vi "Create Dataset.vi"(7 "Dims meas":u64[](array[numeric]), 8 "error in (no error)":errorcluster, 9 "Variant":variant, 10 "Label.Text":string, 11 "Refnum in":T1) -> (0 "error out":errorcluster, 3 "Refnum out":T1)   [LabVIEW 2019]
uses:
  <vilib>/UPVI/lvhdf5/library.llb/HDF5 Ref.ctl
  <vilib>/Utility/Data Type/Type Definitions/Data Type.ctl
  <vilib>/UPVI/lvhdf5/property.llb/LVH5PClassId.ctl
  <vilib>/UPVI/lvhdf5/datatype.llb/LVH5Tcreate_element_type (Variant).vi
  <vilib>/UPVI/lvhdf5/datatype.llb/LVH5Tcreate_dataset_type (Variant).vi
  <vilib>/UPVI/lvhdf5/datatype.llb/LVH5Tcreate_element_type.xnode
  <vilib>/UPVI/lvhdf5/datatype.llb/LVH5Tcreate_dataset_type.xnode
  <vilib>/Utility/Data Type/NI_Data Type.lvlib
panel:
  out "Dims nat":u64[](array[numeric])
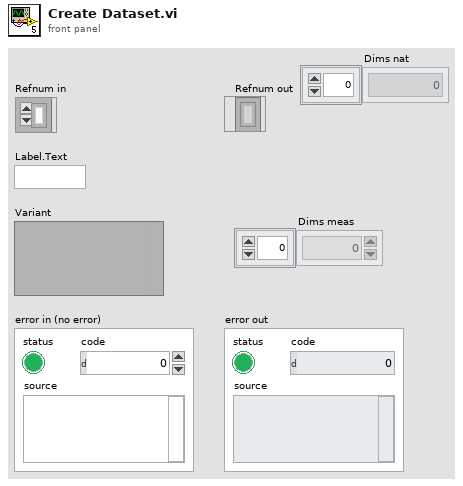
[diagram p1: front panel]
types:
  T1 = typedef "HDF5 Ref.ctl" = refnum<k1>
  T2 = typedef "LVH5PClassId.ctl" = enum32{"H5P_ROOT", "H5P_OBJECT_CREATE", "H5P_FILE_CREATE", "H5P_FILE_ACCESS", "H5P_DATASET_CREATE", "H5P_DATASET_ACCESS", "H5P_DATASET_XFER", "H5P_FILE_MOUNT", "H5P_GROUP_CREATE", "H5P_GROUP_ACCESS", "H5P_DATATYPE_CREATE", "H5P_DATATYPE_ACCESS", "H5P_STRING_CREATE", "H5P_ATTRIBUTE_CREATE", "H5P_OBJECT_COPY", "H5P_LINK_CREATE", "H5P_LINK_ACCESS"}
  T3 = typedef "NI_Data Type.lvlib/Data Type.ctl" = enum8{"Invalid Type", "Void", "I8", "I16", "I32", "I64", "U8", "U16", "U32", "U64", "Single Float", "Double Float", "Extended Float", "Single Complex", "Double Complex", "Extended Complex", "Enum U8", "Enum U16", "Enum U32", "Enum U64", "Single Float With Unit", "Double Float With Unit", "Extended Float With Unit", "Single Complex with Unit", "Double Complex with Unit", "Extended Complex with Unit", "Boolean", "String", "Path", "Picture", "Tag", "Array", "Cluster", "Variant", "LV Variant", "Waveform", "Timestamp", "Digital Waveform", "Digital Data", "ExpressData", "Refnum", "External Data", "VI", "Poly VI", "LabVIEW Class Instance", "Fixed Point", "Set Collection", "Map Collection"}
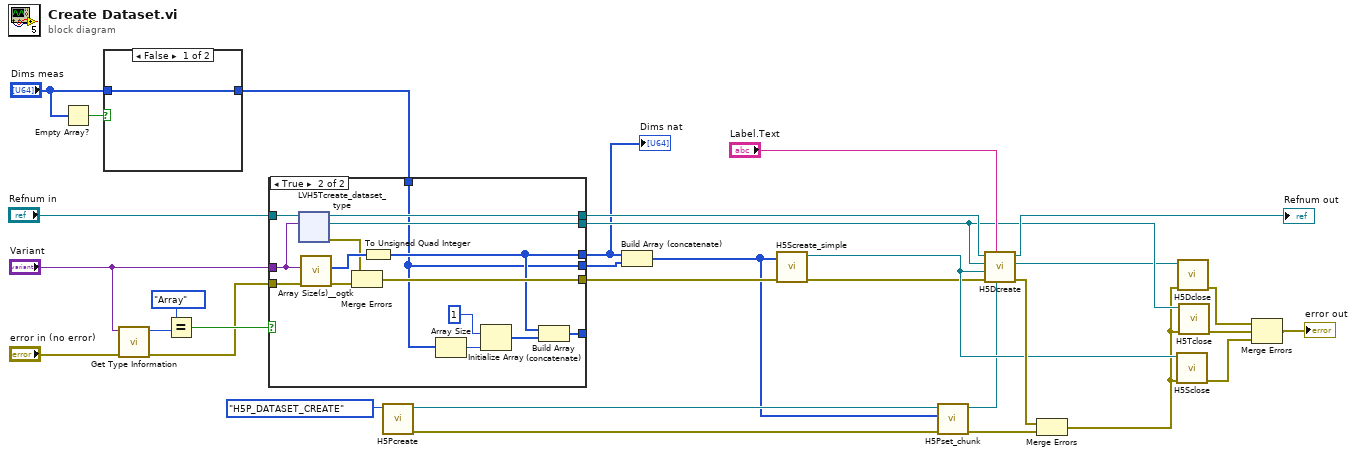
[diagram p0: block diagram]
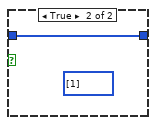
[diagram p2: hidden frame]
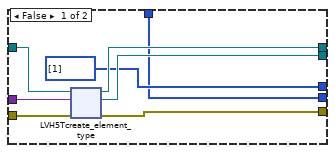
[diagram p3: hidden frame]
diagram:
  n1 = Empty Array?(array="Dims meas") -> (empty?=w4:bool)
  n2 = case shown="False" w4 {
    tunnel: "Dims meas" -> [w33 w34]
    tunnel: [w33 w34] -> w3
    frame False {
    }
    frame True {
      (unwired) u64[] [1] ("Dims meas")
    }
  }
  n3 = call <vilib>:"Get Type Information.vi"("error in (no error)"="error in (no error)", "variant"="Variant") -> ("error out"=w25:errorcluster, "type"=w30:T3)  [unwired: 5 in, 3 out]
  n4 = Equal?(x=Data_Type."Array", y=w30) -> (x = y?=w28:bool)
  n5 = case shown="True" w28 {
    tunnel: "Variant" -> [w37 w77]
    tunnel: w25 -> [w42 w81]
    tunnel: [u64[] [1] w72] -> w8
    tunnel: [w41 w76] -> w22
    tunnel: "Refnum in" -> [w40 w78]
    tunnel: [w38 w74] -> w20
    tunnel: [w39 w73] -> w23
    tunnel: [_ w71] -> _
    tunnel: w3 -> [w35 w67]
    tunnel: [w35 w67] -> w1
    frame False {
      n6 = xnode "LVH5Tcreate_element_type"("HDF5 Location Ref"=w40, "error in (no error)"=w42, "Data"=w37) -> ("HDF5 Location Ref out"=w39:T1, "HDF5 Type Ref"=w38:T1, "error out"=w41:errorcluster)  [unwired: 3 in, 2 out]
    }
    frame True {
      n7 = xnode "LVH5Tcreate_dataset_type"("HDF5 Location Ref"=w78, "Data"=w77) -> ("HDF5 Location Ref out"=w73:T1, "HDF5 Type Ref"=w74:T1, "error out"=w75:errorcluster)  [unwired: 4 in, 2 out]
      n8 = call <userlib>:"Array Size(s)__ogtk.vi"("error in (no error)"=w81, "Array"=w77) -> ("error out"=w79:errorcluster, "Size(s)"=w80:u32[])  [unwired: 7 in, 1 out]
      n9 = Merge Errors(w75, w79) -> (w76:errorcluster)
      n10 = To Unsigned Quad Integer(1:w80) -> (0:w72:u64[])
      n11 = Array Size(array=w67) -> (size(s)=w69:i32)
      n12 = Initialize Array(u64 1 ("element"), w69) -> (w70:u64[])
      n13 = Build Array (concatenate)(w72, w70) -> (w71:u64[])
    }
  }
  "Dims nat" <- w8
  n14 = call <vilib>:"H5Pcreate.vi"("Property List Class"=LVH5PClassId."H5P_DATASET_CREATE") -> ("error out"=w7:errorcluster, "HDF5 Property List Ref"=w6:T1)  [unwired: 7 in]
  n15 = Build Array (concatenate)(w8, w1) -> (w2:u64[])
  n16 = call <vilib>:"H5Screate_simple.vi"("error in (no error)"=w22, "Dimensions"=w2) -> ("error out"=w17:errorcluster, "HDF5 Ref out"=w18:T1)  [unwired: 6 in]
  n17 = call <vilib>:"H5Pset_chunk.vi"("error in (no error)"=w7, "Dimensions"=w2, "HDF5 Property Ref"=w6) -> ("error out"=w15:errorcluster, "HDF5 Ref out"=w16:T1)  [unwired: 5 in]
  n18 = call <vilib>:"H5Dcreate.vi"("Dataset Creation Property List"=w16, "Name"="Label.Text", "error in (no error)"=w17, "HDF5 Dataspace Ref"=w18, "HDF5 Datatype Ref"=w20, "HDF5 Location Ref"=w23) -> ("error out"=w21:errorcluster, "HDF5 Dataset Ref"=w19:T1, "HDF5 Ref out"=→"Refnum out":T1)  [unwired: 3 in]
  n19 = Merge Errors(w21, w15) -> (w14:errorcluster)
  n20 = call <vilib>:"H5Sclose.vi"("error in (no error)"=w14, "HDF5 Dataspace Ref"=w18) -> ("error out"=w11:errorcluster)  [unwired: 7 in]
  n21 = call <vilib>:"H5Dclose.vi"("error in (no error)"=w14, "HDF5 Dataset Ref"=w19) -> ("error out"=w13:errorcluster)  [unwired: 7 in]
  n22 = call <vilib>:"H5Tclose.vi"("error in (no error)"=w14, "HDF5 Datatype Ref"=w20) -> ("error out"=w12:errorcluster)  [unwired: 7 in]
  n23 = Merge Errors(w13, w12, w11) -> (→"error out":errorcluster)
